vi "Zoom to Fit.vi"(8 "error in":errorcluster, 11 "BigMAQ in":refnum<class "BigMAQ.lvclass">) -> (0 "error out":errorcluster, 1 "ZoomSingle":cluster{"X":sgl, "Y":sgl}, 3 "BigMAQ out":refnum<class "BigMAQ.lvclass">)   [LabVIEW 2019, in "BigMAQ.lvclass"]
uses:
  BigMAQ.lvclass
  BigMAQ.lvclass/BigMAQ.ctl
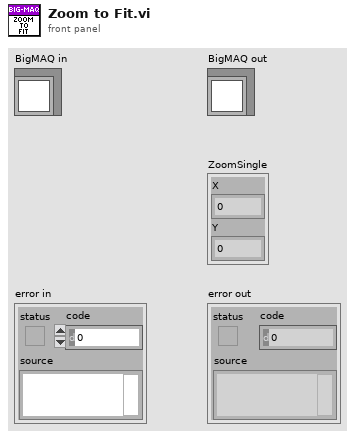
[diagram p1: front panel]
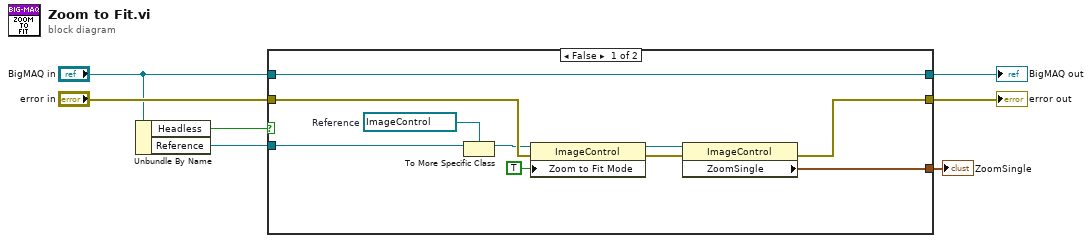
[diagram p0: block diagram]
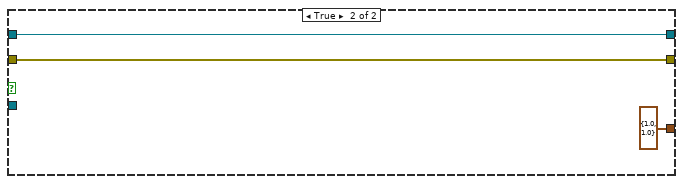
[diagram p2: hidden frame]
diagram:
  n1 = Unbundle By Name("BigMAQ in") -> ("Headless"=w2:bool, "Reference"=w7:refnum<vi>)
  n2 = case shown="False" w2 {
    tunnel: w7 -> [w10 _]
    tunnel: "error in" -> [w16 w19]
    tunnel: [w12 w19] -> w5
    tunnel: "BigMAQ in" -> [w15 w20]
    tunnel: [w15 w20] -> w3
    tunnel: [w11 cluster{"X":sgl, "Y":sgl} {"X"=1.0, "Y"=1.0} ("ZoomSingle")] -> w1
    frame False {
      w9 = refnum<vi> refnum  # Reference
      n3 = To More Specific Class(target class=w9, reference=w10) -> (specific class reference=w8:refnum<vi>)  [unwired: 1 in, 1 out]
      n4 = property class="ImageControl"(reference=w8, error in=w16, "Zoom to Fit Mode"=TRUE) -> (reference out=w14:refnum<vi>, error out=w13:errorcluster)
      n5 = property class="ImageControl"(reference=w14, error in=w13) -> (error out=w12:errorcluster, "ZoomSingle"=w11:cluster{"X":sgl, "Y":sgl})  [unwired: 1 out]
    }
    frame True {
    }
  }
  "error out" <- w5
  "BigMAQ out" <- w3
  "ZoomSingle" <- w1
